vi "Measure Edges.vi"() -> ()   [LabVIEW 2020]
panel:
  in  "Calib path":path
  out "error out":errorcluster
  in  "error in (no error)":errorcluster
  in  "Image Path":path=path "C:/Users/Dell/Documents/Sistemi di visione/ProgrammiCompleti/Image/sd.jpeg"
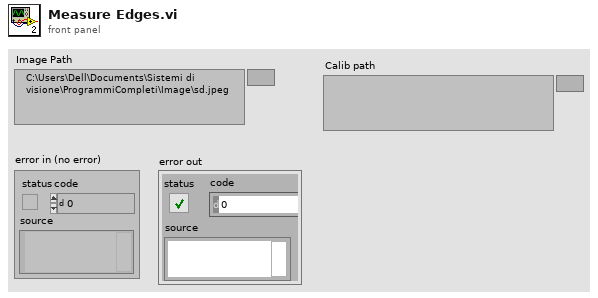
[diagram p1: front panel]
types:
  T1 = typedef "IMAQ Image.ctl" = refnum<image>
  T2 = typedef "Edge New.ctl" = cluster{"Location (Pixel)":cluster{"X":sgl, "Y":sgl}, "Location (Real-World)":cluster{"X":sgl, "Y":sgl}, "Distance (Pixel)":dbl, "Distance (Real-World)":dbl, "Strength":dbl, "Noise":dbl, "Rising?":bool}
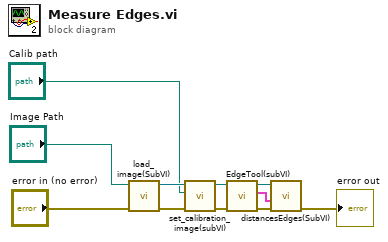
[diagram p0: block diagram]
diagram:
  n1 = call "load_image(SubVI).vi"("error in (no error)"="error in (no error)", "Image Path"="Image Path") -> ("error out"=w3:errorcluster, "Image GRAY"=w5:T1)  [unwired: 8 in]
  n2 = call "set_calibration_image(subVI).vi"("error in (no error)"=w3, "File Path"="Calib path", "Image Dst"=w5) -> ("error out"=w1:errorcluster, "Image Out"=w2:T1)  [unwired: 6 in, 1 out]
  n3 = call "EdgeTool(subVI).vi"("error in (no error)"=w1, "New Image"=w2) -> ("error out"=w6:errorcluster, "Edge Information"=w7:T2[], "Image Out"=w8:T1)  [unwired: 5 in]
  n4 = call "distancesEdges(SubVI).vi"("error in (no error)"=w6, "Edge Information"=w7, "Image In"=w8) -> ("error out"=→"error out":errorcluster)  [unwired: 8 in]
